vi "runtest Parse Step Parameters.vi"(4 "Files Found?":bool, 6 "Instruments on Station":T2[](array[typedef]), 8 "Sequence Count (0)":i32, 9 "Quickmode? (f)":bool, 10 "Step Tab (\"\")":string, 11 "Step Number (0)":i32) -> (3 "Step parameters":T1={"Quick Mode (T)"=FALSE, "Seq Count"=0, "Step Info"="", "Instruments on Station"=[], "LANGUAGE"="English", "Files Found?"=FALSE, "Step Number"=1} {"Step Number" min=1 step=1})   [LabVIEW 2011]
uses:
  server/database/Stations/Instruments/Instrument Record.ctl
  tests/Test Execution Settings.ctl
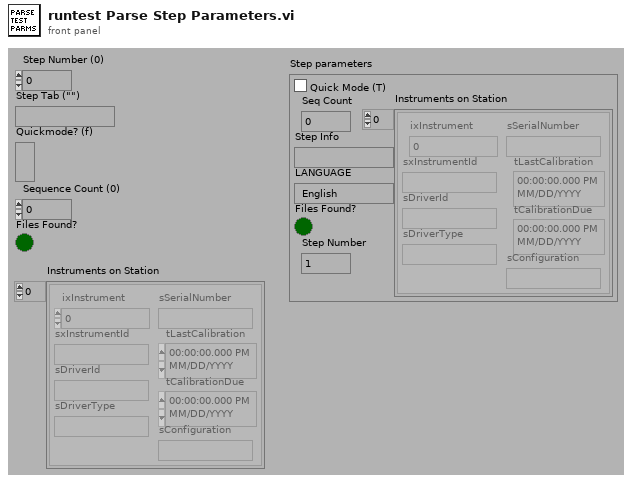
[diagram p1: front panel]
types:
  T1 = typedef "Test Execution Settings.ctl" = cluster{"Quick Mode (T)":bool, "Seq Count":i32, "Step Info":string, "Instruments on Station":T2[], "LANGUAGE":string, "Files Found?":bool, "Step Number":i32}
  T2 = typedef "Instrument Record.ctl" = cluster{"ixInstrument":i32, "sxInstrumentId":string, "sDriverId":string, "sDriverType":string, "sSerialNumber":string, "tLastCalibration":timestamp, "tCalibrationDue":timestamp, "sConfiguration":string}
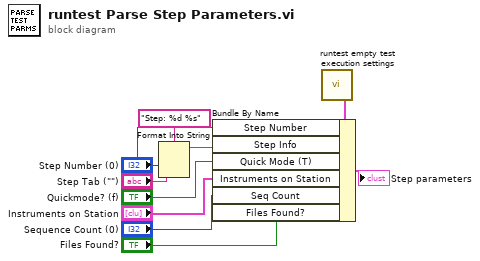
[diagram p0: block diagram]
diagram:
  n1 = Format Into String(format string="Step: %d %s", "Step Number (0)", "Step Tab (\"\")") -> (resulting string=w9:string)  [unwired: 2 in, 1 out]
  n2 = call "runtest empty test execution settings.vi"() -> ("empty Test Execution Settings"=w8:T1)
  n3 = Bundle By Name(cluster=w8, "Step Number"="Step Number (0)", "Step Info"=w9, "Quick Mode (T)"="Quickmode? (f)", "Instruments on Station"="Instruments on Station", "Seq Count"="Sequence Count (0)", "Files Found?"="Files Found?") -> (→"Step parameters":T1)
